vi "Enable Plot (SubVI).vi"(0 "Enable Ref":refnum<vi>, 7 "Strain Chart Ref":refnum<vi>, 13 "Weight Refs":refnum<vi>[](array[refnum])) -> ()   [LabVIEW 2010]
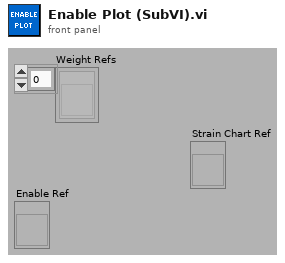
[diagram p1: front panel]
types:
  T1 = enum8{"Enabled", "Disabled", "Disabled and Grayed Out"}
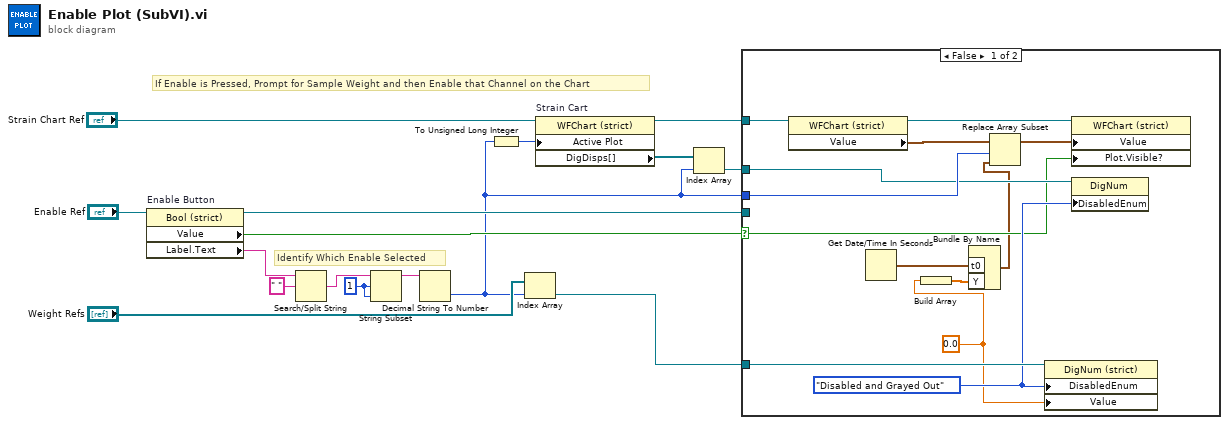
[diagram p0: block diagram]
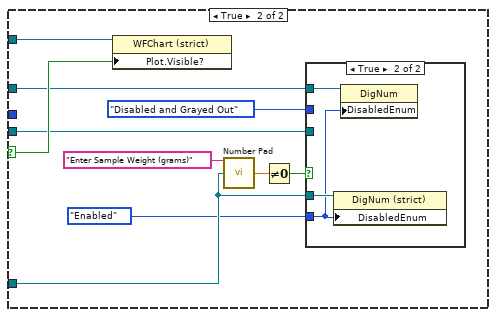
[diagram p2: hidden frame]
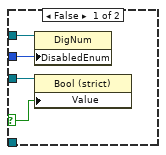
[diagram p3: hidden frame]
diagram:
  w11 = 1
  # "If Enable is Pressed, Prompt for Sample Weight and then Enable that Channel on the Chart"
  # "Identify Which Enable Selected"
  n1 = property on="Enable Button" class="Bool (strict)"(reference="Enable Ref") -> (reference out=w5:refnum<vi>, "Value"=w7:bool, "Label.Text"=w12:string)  [unwired: 1 in, 1 out]
  n2 = Search/Split String(string=w12, search string/char (-)=" ") -> (match + rest of string=w10:string)  [unwired: 1 in, 2 out]
  n3 = String Subset(string=w10, offset (0)=w11, length (rest)=w11) -> (substring=w9:string)
  n4 = Decimal String To Number(string=w9) -> (number=w3:i32)  [unwired: 2 in, 1 out]
  n5 = To Unsigned Long Integer(number=w3) -> (unsigned 32bit integer=w4:u32)
  n6 = Index Array(array="Weight Refs", index=w3) -> (element=w2:refnum<vi>)
  n7 = property on="Strain Cart" class="WFChart (strict)"(reference="Strain Chart Ref", "Active Plot"=w4) -> (reference out=w14:refnum<vi>, "DigDisps[]"=w15:refnum<vi>[])  [unwired: 1 in, 1 out]
  n8 = Index Array(array=w15, index=w3) -> (element=w16:refnum<vi>)
  n9 = case shown="False" w7 {
    selector: w7 -> [w23 w34]
    tunnel: w2 -> [w29 w36]
    tunnel: w14 -> [w27 w35]
    tunnel: w16 -> [w25 w30]
    tunnel: w3 -> [w26 _]
    tunnel: w5 -> [_ w32]
    frame False {
      w19 = 0.0
      w24 = T1."Disabled and Grayed Out" ("Disabled")
      n10 = property class="WFChart (strict)"(reference=w27) -> (reference out=w28:refnum<vi>, "Value"=w22:waveform(dbl)[])  [unwired: 1 in, 1 out]
      n11 = Get Date/Time In Seconds() -> (seconds since 1Jan1904=w21:timestamp)
      n12 = Build Array(w19) -> (w20:dbl[])
      n13 = Bundle By Name("t0"=w21, "Y"=w20) -> (w18:waveform(dbl))  [unwired: 1 in]
      n14 = Replace Array Subset(array=w22, new element=w18, index=w26) -> (w17:waveform(dbl)[])
      n15 = property class="DigNum (strict)"(reference=w29, "DisabledEnum"=w24, "Value"=w19) -> ()  [unwired: 1 in, 2 out]
      n16 = property class="WFChart (strict)"(reference=w28, "Value"=w17, "Plot.Visible?"=w23) -> ()  [unwired: 1 in, 2 out]
      n17 = property class="DigNum"(reference=w25, "DisabledEnum"=w24) -> ()  [unwired: 1 in, 2 out]
    }
    frame True {
      n18 = property class="WFChart (strict)"(reference=w35, "Plot.Visible?"=w34) -> ()  [unwired: 1 in, 2 out]
      n19 = call "Number Pad.vi"("Instruction"="Enter Sample Weight (grams)", "CtlRef"=w36) -> ("Numeric"=w38:dbl)  [unwired: 11 in, 2 out]
      n20 = Not Equal To 0?(x=w38) -> (x != 0?=w37:bool)
      n21 = case shown="True" w37 {
        selector: w37 -> [w42 _]
        tunnel: w36 -> [_ w46]
        tunnel: T1."Enabled" ("Disabled") -> [_ w44]
        tunnel: w32 -> [w43 _]
        tunnel: T1."Disabled and Grayed Out" ("Disabled") -> [w40 _]
        tunnel: w30 -> [w41 w45]
        frame False {
          n22 = property class="DigNum"(reference=w41, "DisabledEnum"=w40) -> ()  [unwired: 1 in, 2 out]
          n23 = property class="Bool (strict)"(reference=w43, "Value"=w42) -> ()  [unwired: 1 in, 2 out]
        }
        frame True {
          n24 = property class="DigNum (strict)"(reference=w46, "DisabledEnum"=w44) -> ()  [unwired: 1 in, 2 out]
          n25 = property class="DigNum"(reference=w45, "DisabledEnum"=w44) -> ()  [unwired: 1 in, 2 out]
        }
      }
    }
  }
